vi "Load_Subpanel.vi"(0 "Sub VI Ref In":refnum<vi>, 1 "SubPanel Ref":refnum<vi>, 2 "Device Handle":i32, 3 "Error In":errorcluster, 4 "VI Path":path) -> (5 "Sub VI Ref Out":refnum<vi>, 7 "Error Out":errorcluster)   [LabVIEW 2014]
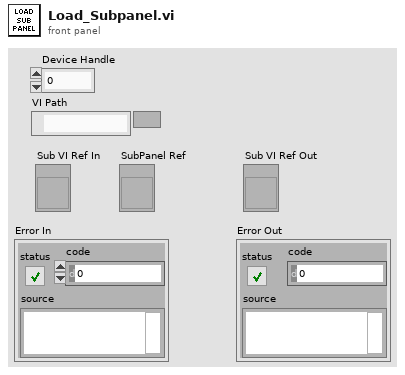
[diagram p1: front panel]
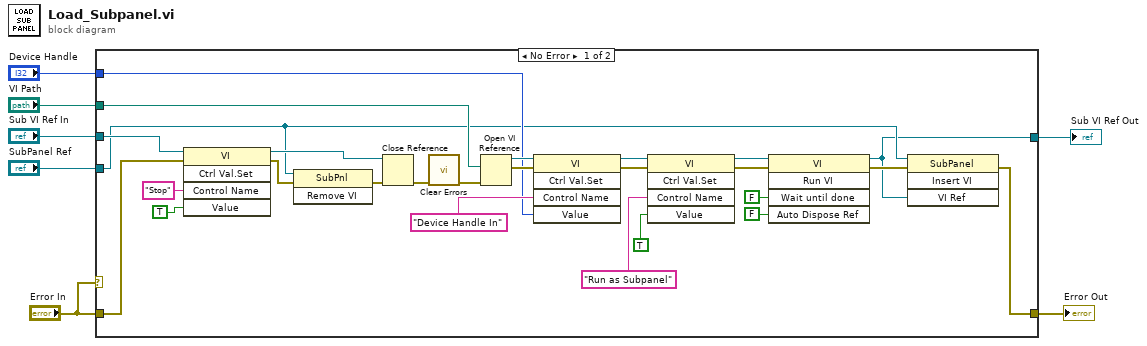
[diagram p0: block diagram]
diagram:
  n1 = case shown="No Error" "Error In" {
    tunnel: "Error In" -> [w13 w34]
    tunnel: "Device Handle" -> [w15 _]
    tunnel: "VI Path" -> [w14 _]
    tunnel: [w12 w34] -> w4
    tunnel: "Sub VI Ref In" -> [w11 _]
    tunnel: "SubPanel Ref" -> [w9 _]
    tunnel: [w8 _] -> w1
    frame No Error {
      n2 = invoke class="VI" method="Ctrl Val.Set"(reference=w11, error in=w13, "Control Name"="Stop", "Value"=TRUE) -> (reference out=w10:refnum<vi>, error out=w33:errorcluster)  [unwired: 1 in, 3 out]
      n3 = invoke on="Invoke Node" class="SubPnl" method="Remove VI"(reference=w9, error in=w33) -> (error out=w30:errorcluster)  [unwired: 1 in, 2 out]
      n4 = Close Reference(reference=w10, error in (no error)=w30) -> (error out=w27:errorcluster)
      n5 = call <vilib>:"Clear Errors.vi"("error in (no error)"=w27) -> ("error out"=w28:errorcluster)  [unwired: 5 in, 1 out]
      n6 = Open VI Reference(vi path=w14, error in (no error)=w28) -> (vi reference=w29:refnum<vi>, error out=w19:errorcluster)  [unwired: 4 in]
      n7 = invoke class="VI" method="Ctrl Val.Set"(reference=w29, error in=w19, "Control Name"="Device Handle In", "Value"=w15) -> (reference out=w21:refnum<vi>, error out=w20:errorcluster)  [unwired: 1 in, 3 out]
      n8 = invoke class="VI" method="Ctrl Val.Set"(reference=w21, error in=w20, "Control Name"="Run as Subpanel", "Value"=TRUE) -> (reference out=w22:refnum<vi>, error out=w25:errorcluster)  [unwired: 1 in, 3 out]
      n9 = invoke class="VI" method="Run VI"(reference=w22, error in=w25, "Wait until done"=FALSE ("Wait Until Done"), "Auto Dispose Ref"=FALSE ("Auto Dispose Reference")) -> (reference out=w8:refnum<vi>, error out=w26:errorcluster)  [unwired: 1 in, 3 out]
      n10 = invoke on="Invoke Node" class="SubPanel" method="Insert VI"(reference=w9, error in=w26, "VI Ref"=w8) -> (error out=w12:errorcluster)  [unwired: 1 in, 3 out]
    }
    frame Error {
    }
  }
  "Error Out" <- w4
  "Sub VI Ref Out" <- w1
